vi "TreeStatic.vi"() -> ()   [LabVIEW 2011]
panel:
  out "String":string
  in  "Tree":string(tree)="李某"
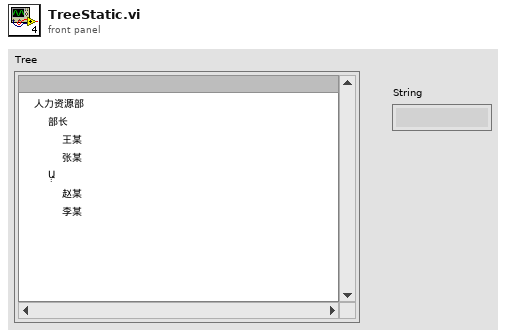
[diagram p1: front panel]
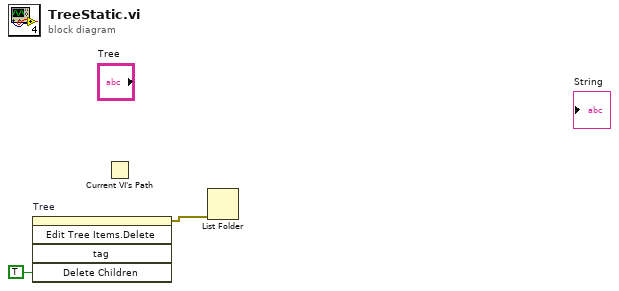
[diagram p0: block diagram]
diagram:
  n1 = invoke on="Tree" class="Tree (strict)" method="Edit Tree Items.Delete"("Delete Children"=TRUE ("Delete Children?")) -> (error out=w1:errorcluster)  [unwired: 4 in, 4 out]
  n2 = Current VI's Path() -> ()  [unwired: 1 out]
  n3 = List Folder(error in=w1) -> ()  [unwired: 3 in, 4 out]
